vi "ROI_FromFirstFrame.vi"(8 "error in":errorcluster, 11 "Image to get ROI":path) -> (0 "error out":errorcluster, 1 "ROI Found?":bool, 2 "ROI":T3 {"Contours"."Type" items=["No Selection", "Point", "Line", "Rectangle", "Oval", "Polygon", "Freehand Region", "Annulus", "Unused2", "Unused3", "Broken Line", "Freehand Line", "Rotated Rectangle"]}, 3 "ROI Out (U8)":T2, 4 "LIMLOCALMETADATA":T1, 5 "Original Image (I16)":T2)   [LabVIEW 2012]
uses:
  <vilib>/vision/Image Controls.llb/IMAQ Image.ctl
  ND2_Reader_32bit/controls/cluster_LIMLOCALMETADATA.ctl
  FileIO/TypeDef - File Actions.ctl
  <vilib>/vision/NI_Vision_Development_Module.lvlib
  ND2_Reader_32bit/ND2_Reader_32.lvlib
panel:
  out "Image Display":T2(plugin-control)
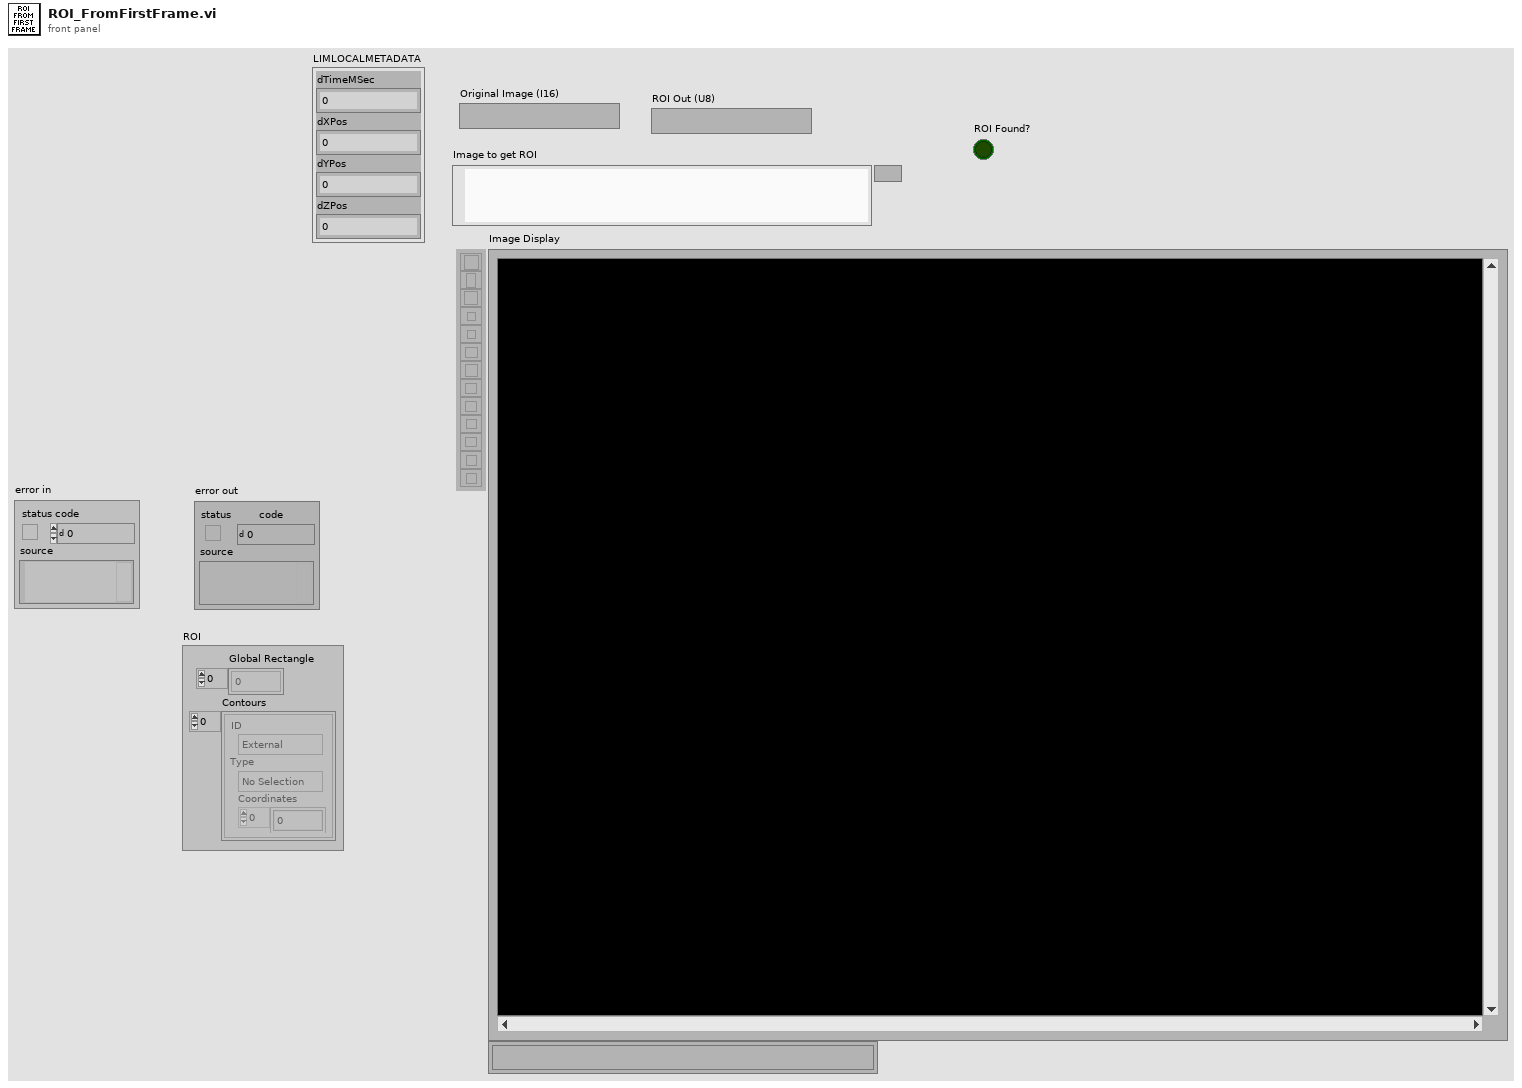
[diagram p1: front panel]
types:
  T1 = typedef "cluster_LIMLOCALMETADATA.ctl" = cluster{"dTimeMSec":dbl, "dXPos":dbl, "dYPos":dbl, "dZPos":dbl}
  T2 = typedef "IMAQ Image.ctl" = refnum<image>
  T3 = typedef "ROI Descriptor" = cluster{"Global Rectangle":i32[], "Contours":cluster{"ID":enum32{"External", "Internal"}, "Type":u32, "Coordinates":i32[]}[]}
  T4 = cluster{"Measurement Parameter":i32, "Range Lower Value":dbl, "Range Upper Value":dbl, "Range":bool, "Measurement Type":bool}
  T5 = typedef "TypeDef - File Actions.ctl" = enum16{"Read", "Write", "Get Current"}
  T6 = typedef "Image Type" = u32
  T7 = typedef "TypeDef - System Configuration.ctl" = cluster{"Results FilePath":path, "Analysis Parameters":cluster{"Threshold Range":cluster{"Lower Value":i32, "Upper Value":i32}, "Particle Erosion":cluster{"N Steps":u32}, "Feret Filter ":cluster{"Lower Value":dbl, "Upper Value":dbl}, "Circle Filter Diameter":cluster{"Min Radius":sgl, "Max Radius":sgl}}}
  T8 = cluster{"Measurement Parameter":i32, "Range Lower Value":dbl, "Range Upper Value":dbl, "Range":bool, "Measurement Type":bool}[]
  T9 = cluster{"Pos. X":i32, "Pos. Y":i32, "Radius":i32, "Core Area":i32}[]
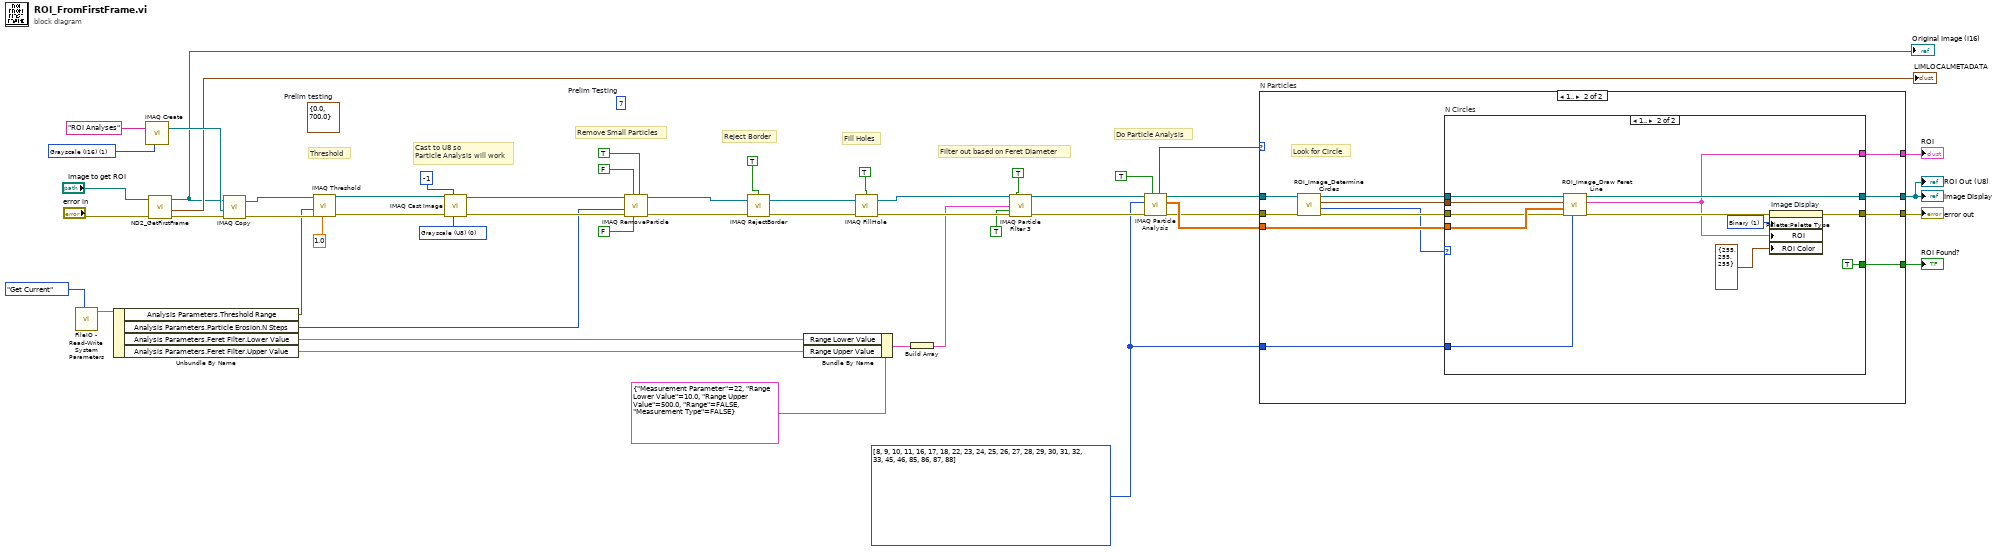
[diagram p0: block diagram]
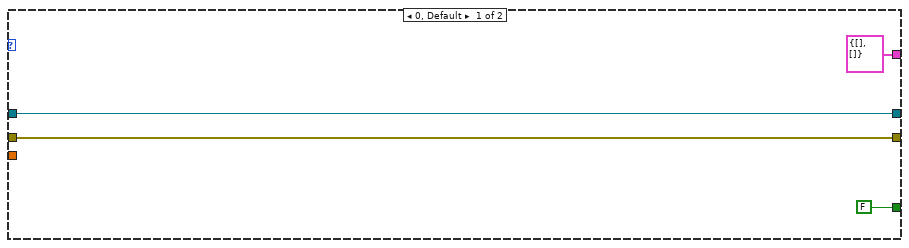
[diagram p2: hidden frame]
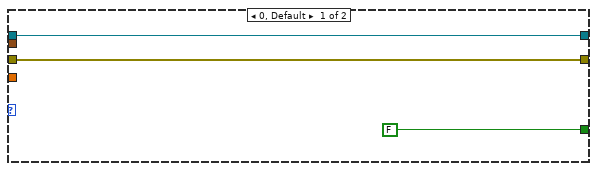
[diagram p3: hidden frame]
diagram:
  w16 = T6 1 items=["Grayscale (U8)", "Grayscale (I16)", "Grayscale (SGL)", "Complex (CSG)", "RGB (U32)", "HSL (U32)", "RGB (U64)", "Grayscale (U16)"] ("Image Type")
  w34 = i32[] [8, 9, 10, 11, 16, 17, 18, 22, 23, 24, 25, 26, 27, 28, 29, 30, 31, 32, 33, 45, 46, 85, 86, 87, 88] items=["Center of Mass X", "Center of Mass Y", "First Pixel X", "First Pixel Y", "Bounding Rect Left", "Bounding Rect Top", "Bounding Rect Right", "Bounding Rect Bottom", "Max Feret Diameter Start X", "Max Feret Diameter Start Y", "Max Feret Diameter End X", "Max Feret Diameter End Y", "Max Horiz. Segment Length Left", "Max Horiz. Segment Length Right", "Max Horiz. Segment Length Row", "-", "Bounding Rect Width", "Bounding Rect Height", "Bounding Rect Diagonal", "Perimeter", "Convex Hull Perimeter", "Holes' Perimeter", "Max Feret Diameter", "Equivalent Ellipse Major Axis", "Equivalent Ellipse Minor Axis", "Equivalent Ellipse Minor Axis (Feret)", "Equivalent Rect Long Side", "Equivalent Rect Short Side", "Equivalent Rect Diagonal", "Equivalent Rect Short Side (Feret)", "Average Horiz. Segment Length", "Average Vert. Segment Length", "Hydraulic Radius", "Waddel Disk Diameter", "-", "Area", "Holes' Area", "Particle & Holes' Area", "Convex Hull Area", "Image Area", "-", "Number of Holes", "Number of Horiz. Segments", "Number of Vert. Segments", "-", "Orientation", "Max Feret Diameter Orientation", "-", "% Area/Image Area", "% Area/(Particle & Holes' Area)", "Ratio of Equivalent Ellipse Axes", "Ratio of Equivalent Rect Sides", "-", "Elongation Factor", "Compactness Factor", "Heywood Circularity Factor", "Type Factor", "-", "Sum X", "Sum Y", "Sum XX", "Sum XY", "Sum YY", "Sum XXX", "Sum XXY", "Sum XYY", "Sum YYY", "-", "Moment of Inertia XX", "Moment of Inertia XY", "Moment of Inertia YY", "Moment of Inertia XXX", "Moment of Inertia XXY", "Moment of Inertia XYY", "Moment of Inertia YYY", "Norm. Moment of Inertia XX", "Norm. Moment of Inertia XY", "Norm. Moment of Inertia YY", "Norm. Moment of Inertia XXX", "Norm. Moment of Inertia XXY", "Norm. Moment of Inertia XYY", "Norm. Moment of Inertia YYY", "Hu Moment 1", "Hu Moment 2", "Hu Moment 3", "Hu Moment 4", "Hu Moment 5", "Hu Moment 6", "Hu Moment 7"] ("Pixel Measurements")
  (unwired) 7  # Prelim Testing
  w49 = T6 0 items=["Grayscale (U8)", "Grayscale (I16)", "Grayscale (SGL)", "Complex (CSG)", "RGB (U32)", "HSL (U32)", "RGB (U64)", "Grayscale (U16)"] ("Image Type")
  (unwired) cluster{"Lower value":sgl, "Upper value":sgl} {"Lower value"=0.0, "Upper value"=700.0}  # Prelim testing
  # "Do Particle Analysis"
  # "Fill Holes"
  # "Reject Border"
  # "Remove Small Particles"
  # "Filter out based on Feret Diameter"
  # "Cast to U8 so \nParticle Analysis will work"
  # "Threshold"
  n1 = call "FileIO - Read-Write System Parameters.vi"("Action"=TypeDef_-_File_Actions."Get Current") -> ("HW Configuration (each Station)"=w8:T7)  [unwired: 9 in, 1 out]
  n2 = Unbundle By Name(w8) -> ("Analysis Parameters.Threshold Range"=w7:cluster{"Lower Value":i32, "Upper Value":i32}, "Analysis Parameters.Particle Erosion.N Steps"=w6:u32, "Analysis Parameters.Feret Filter.Lower Value"=w4:dbl, "Analysis Parameters.Feret Filter.Upper Value"=w3:dbl)
  n3 = call "IMAQ Create"("Image Name"="ROI Analyses", "Image Type"=w16) -> ("New Image"=w13:T2)  [unwired: 3 in, 1 out]
  n4 = call "ND2_GetFirstFrame.vi"("error in (no error)"="error in", "FilePath"="Image to get ROI") -> ("error out"=w15:errorcluster, "LIMLOCALMETADATA"=→"LIMLOCALMETADATA":T1, "Image out"=w10:T2)  [unwired: 7 in]
  "Original Image (I16)" <- w10
  n5 = call "IMAQ Copy"("error in (no error)"=w15, "Image Dst"=w13, "Image Src"=w10) -> ("error out"=w14:errorcluster, "Image Dst Out"=w12:T2)  [unwired: 3 in]
  n6 = call "IMAQ Threshold"("Replace Value"=sgl 1.0, "error in (no error)"=w14, "Range"=w7, "Image Src"=w12) -> ("error out"=w51:errorcluster, "Image Dst Out"=w28:T2)  [unwired: 2 in, 4 out]
  n7 = call "IMAQ Cast Image"("Image Type"=w49, "# Shifts"=-1, "error in (no error)"=w51, "Image Src"=w28) -> ("error out"=w27:errorcluster, "Image Dst Out"=w26:T2)  [unwired: 2 in, 4 out]
  n8 = call "IMAQ RemoveParticle"("Connectivity 4/8 (8)"=TRUE, "Low Pass/High Pass (Low)"=FALSE, "Square/Hexa (Square)"=FALSE, "error in (no error)"=w27, "Number of Erosion"=w6, "Image Src"=w26) -> ("error out"=w45:errorcluster, "Image Dst Out"=w29:T2)  [unwired: 1 in, 3 out]
  n9 = call "IMAQ RejectBorder"("error in (no error)"=w45, "Image Src"=w29, "Connectivity 4/8 (8)"=TRUE) -> ("error out"=w43:errorcluster, "Image Dst Out"=w30:T2)  [unwired: 1 in, 2 out]
  n10 = Bundle By Name(cluster=T4 {"Measurement Parameter"=22, "Range Lower Value"=10.0, "Range Upper Value"=500.0, "Range"=FALSE, "Measurement Type"=FALSE} ("Selection Value"), "Range Lower Value"=w4, "Range Upper Value"=w3) -> (w2:T4)
  n11 = call "IMAQ FillHole"("error in (no error)"=w43, "Image Src"=w30, "Connectivity 4/8 (8)"=TRUE) -> ("error out"=w41:errorcluster, "Image Dst Out"=w32:T2)  [unwired: 1 in, 2 out]
  n12 = Build Array(w2) -> (w1:T8)
  n13 = call "IMAQ Particle Filter 3"("Image Src"=w32, "Connectivity 4/8 (8)"=TRUE, "Selection Values"=w1, "Keep/Remove Particles (F)"=TRUE ("Keep/Remove Particles"), "error in (no error)"=w41) -> ("Image Dst Out"=w33:T2, "error out"=w38:errorcluster)  [unwired: 4 in, 5 out]
  n14 = call "IMAQ Particle Analysis"("Connectivity 4/8 (8)"=TRUE, "error in (no error)"=w38, "Pixel Measurements"=w34, "Image"=w33) -> ("error out"=w21:errorcluster, "Particle Measurements (Pixels)"=w35:dbl[][], "Image Out (duplicate)"=w22:T2, "Number of Particles"=w20:i32)  [unwired: 1 in, 3 out]
  n15 = case "N Particles" shown="1.." w20 {
    tunnel: [w54 w67] -> w36
    tunnel: [w55 w66] -> w18
    tunnel: w35 -> [_ w65]
    tunnel: w34 -> [_ w64]
    tunnel: [T3 {"Global Rectangle"=[], "Contours"=[]} ("ROI") w62] -> w31
    tunnel: w22 -> [w55 w61]
    tunnel: w21 -> [w54 w60]
    tunnel: [FALSE w56] -> w19
    frame 0, Default {
    }
    frame 1.. {
      # "Look for Circle"
      n16 = call "ROI_Image_Determine Circles.vi"("error in (no error)"=w60, "Image in"=w61) -> ("error out"=w63:errorcluster, "N Circles"=w57:i32, "Circle Data"=w58:T9, "Image out"=w59:T2)  [unwired: 6 in]
      n17 = case "N Circles" shown="1.." w57 {
        tunnel: [w70 w81] -> w67
        tunnel: [w69 w80] -> w66
        tunnel: w65 -> [_ w78]
        tunnel: w64 -> [_ w77]
        tunnel: w63 -> [w70 w76]
        tunnel: [_ w75] -> w62
        tunnel: w59 -> [w69 w73]
        tunnel: w58 -> [_ w72]
        tunnel: [FALSE TRUE] -> w56
        frame 0, Default {
        }
        frame 1.. {
          w82 = u32 1 items=["Grayscale", "Binary", "Gradient", "Rainbow", "Temperature", "User Defined"] ("Palette")
          n18 = call "ROI_Image_Draw Feret Line.vi"("Pixel Measurements"=w77, "error in (no error)"=w76, "Particle Measurements (Pixels)"=w78, "Circles Data"=w72, "Image in"=w73) -> ("error out"=w79:errorcluster, "ROI"=w75:T3, "Image out"=w80:T2)  [unwired: 4 in]
          n19 = property on="Image Display" class="ImageControl"(error in=w79, "Palette:Palette Type"=w82, "ROI"=w75, "ROI Color"=cluster{"Red":u8, "Green":u8, "Blue":u8} {"Red"=255, "Green"=255, "Blue"=255}) -> (error out=w81:errorcluster)  [unwired: 1 in, 1 out]
        }
      }
    }
  }
  "error out" <- w36
  "Image Display" <- w18
  "ROI" <- w31
  "ROI Out (U8)" <- w18
  "ROI Found?" <- w19
